vi "server-new.vi"() -> ()   [LabVIEW 2016]
uses:
  <vilib>/rvi/eio/common/nirviEmuClasses.ctl
  <vilib>/rvi/Emulation/niFpgaSctlEmulationGetInTimedLoop.vi
  <vilib>/rvi/Emulation/niFpgaProcessEmulError.vi
  <vilib>/rvi/eio/common/nirviEmuTemplateMethod_errors.vi
  <vilib>/rvi/Emulation/niFpgaEmulationIsFPGAContextNoSignature.vi
  <vilib>/rvi/DataTransferAndStorage/Container/Common/niFpgaContainerGetUniqueNameForEmu.vi
  <vilib>/rvi/Memory/Memory_Emulation/niFpgaMemoryEmulationCacheClearOnFirstRun.vi
  <vilib>/rvi/Memory/Memory_Emulation/nirvimemoryEmulationManagerCache_MakeExclusive.vi
  <vilib>/rvi/Memory/Memory_Emulation/niFpgaMemoryEmulationValidateCache.vi
  <vilib>/rvi/Memory/Memory_Emulation/nirvimemoryEmulationManagerCache_InsertValue.vi
  <vilib>/Utility/error.llb/Clear Errors.vi
  <vilib>/rvi/Memory/Memory_Emulation/nirvimemoryEmulationManagerCache_ReleaseExclusive.vi
  <vilib>/rvi/Memory/Memory_Emulation/nirvimemoryEmulationManagerCache_GetValue.vi
  <vilib>/rvi/Memory/Memory_Emulation/nirvimemoryEmulationManagerCache_SetValue.vi
  <vilib>/rvi/Emulation/niFpgaGetClockAttributes.vi
  <vilib>/rvi/Emulation/niFpgaEmulationReportErrorSimple.vi
  <vilib>/rvi/Emulation/niFpgaCriticalErrorInLSC.vi
  <vilib>/rvi/eio/common/nirviEmuTemplateMethod_noerrors.vi
  <vilib>/rvi/errors/niFpgaSetErrorForExecOnDevCompSimple.vi
  <vilib>/rvi/eio/common/nirviEmuReportErrorAndStop.vi
  <vilib>/rvi/FIFO/Fifo_Resource/nirvififoEmulationSetSize.vi
  <vilib>/rvi/FIFO/Fifo_Resource/nirviFifoEmulationQueueMgr.vi
  <instcachedir>/0/nirviFifoEmulationQueueMgr_E5CAEC123FF24DC58D834DCA3CDAA9B5.lvgen/nirviFifoEmulationQueueMgr_E5CAEC123FF24DC58D834DCA3CDAA9B5_001.vi
  <vilib>/rvi/FIFO/Fifo_Resource/nirvififoEmulationDetermineInputValidOut.vi
  <vilib>/rvi/FIFO/Fifo_Resource/nirvififoEmulationCreateLock.vi
  <vilib>/rvi/FIFO/Fifo_Resource/nirvififoEmulationObtainLock.vi
  <vilib>/rvi/FIFO/Fifo_Resource/nirvififoEmulationReleaseLock.vi
  <vilib>/rvi/occurrence/nirviWaitOnOccurrenceBase.vi
  <vilib>/rvi/errors/nirviReportUnexpectedCaseInternalError.vi
  <vilib>/rvi/errors/nirviReportUnexpectedCaseInternalError (U32).vi
  <vilib>/eio/EIOGrowableMethodNode/genericMethod/EIOGrowableMethodNode.xnode
  <vilib>/rvi/eio/nirviEIOMethodImplementation/nirviEIOMethodImplementation.xnode
  <vilib>/rvi/eio/nirviErrorMerge/nirviErrorMerge.xnode
  <vilib>/rvi/DataTransferAndStorage/Container/XNode/niFpgaContainer.xnode
  <vilib>/rvi/DataTransferAndStorage/Register/Emulation/niFpgaRegisterEmulation.vi
  <vilib>/eio/EIONode/EIONode.xnode
  <vilib>/rvi/FIFO/Fifo_Resource/nirvififoEmulationWrite.vi
panel:
  in  "DO":u32
  in  "Fan Voltage":i16
  out "pas lrms":u32
  out "Temperatures":T1
  out "Sensor Status":u8
  in  "f1":u32
  in  "f0":u32
  in  "Transmit?":bool
  in  "CRDSampData":u32
  in  "Speaker":cluster{"Vscale":fxp<+,32,0>, "Offset":i16}
  in  "Stop":bool
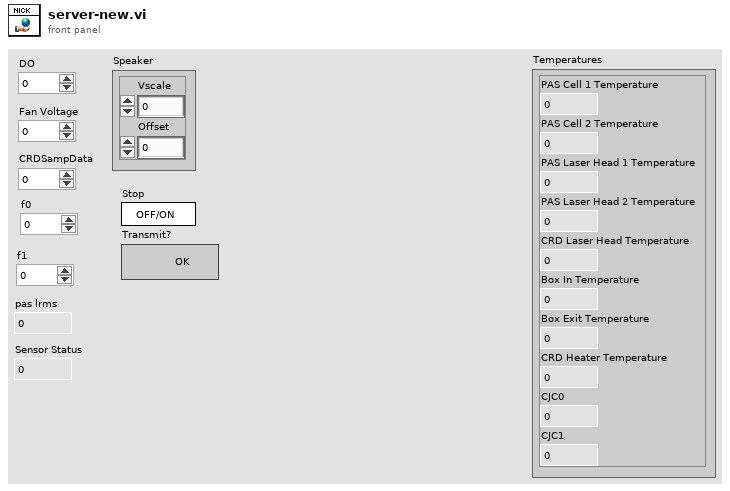
[diagram p1: front panel]
types:
  T1 = cluster{"PAS Cell 1 Temperature":fxp<+/-,24,-2>, "PAS Cell 2 Temperature":fxp<+/-,24,-2>, "PAS Laser Head 1 Temperature":fxp<+/-,24,-2>, "PAS Laser Head 2 Temperature":fxp<+/-,24,-2>, "CRD Laser Head Temperature":fxp<+/-,24,-2>, "Box In Temperature":fxp<+/-,24,-2>, "Box Exit Temperature":fxp<+/-,24,-2>, "CRD Heater Temperature":fxp<+/-,24,-2>, "CJC0":fxp<+/-,24,-2>, "CJC1":fxp<+/-,24,-2>}
  T2 = typedef "nirviEmuClasses.ctl" = enum16{"IO Read", "IO Write", "Method", "Property Read", "Property Write"}
  T3 = cluster{"PAS Cell 1 Temperature":fxp<+/-,24,-2>, "PAS Cell 2 Temperature":fxp<+/-,24,-2>, "PAS Laser Head 1 Temperature":fxp<+/-,24,-2>, "PAS Laser Head 2 Temperature":fxp<+/-,24,-2>, "CRD Laser Head Temperature":fxp<+/-,24,-2>, "Box In Temperature":fxp<+/-,24,-2>, "Box Exit Temperature":fxp<+/-,24,-2>, "CRD Heater Temperature":fxp<+/-,24,-2>, "Mod5/CJC0":fxp<+/-,24,-2>, "Mod5/CJC1":fxp<+/-,24,-2>}
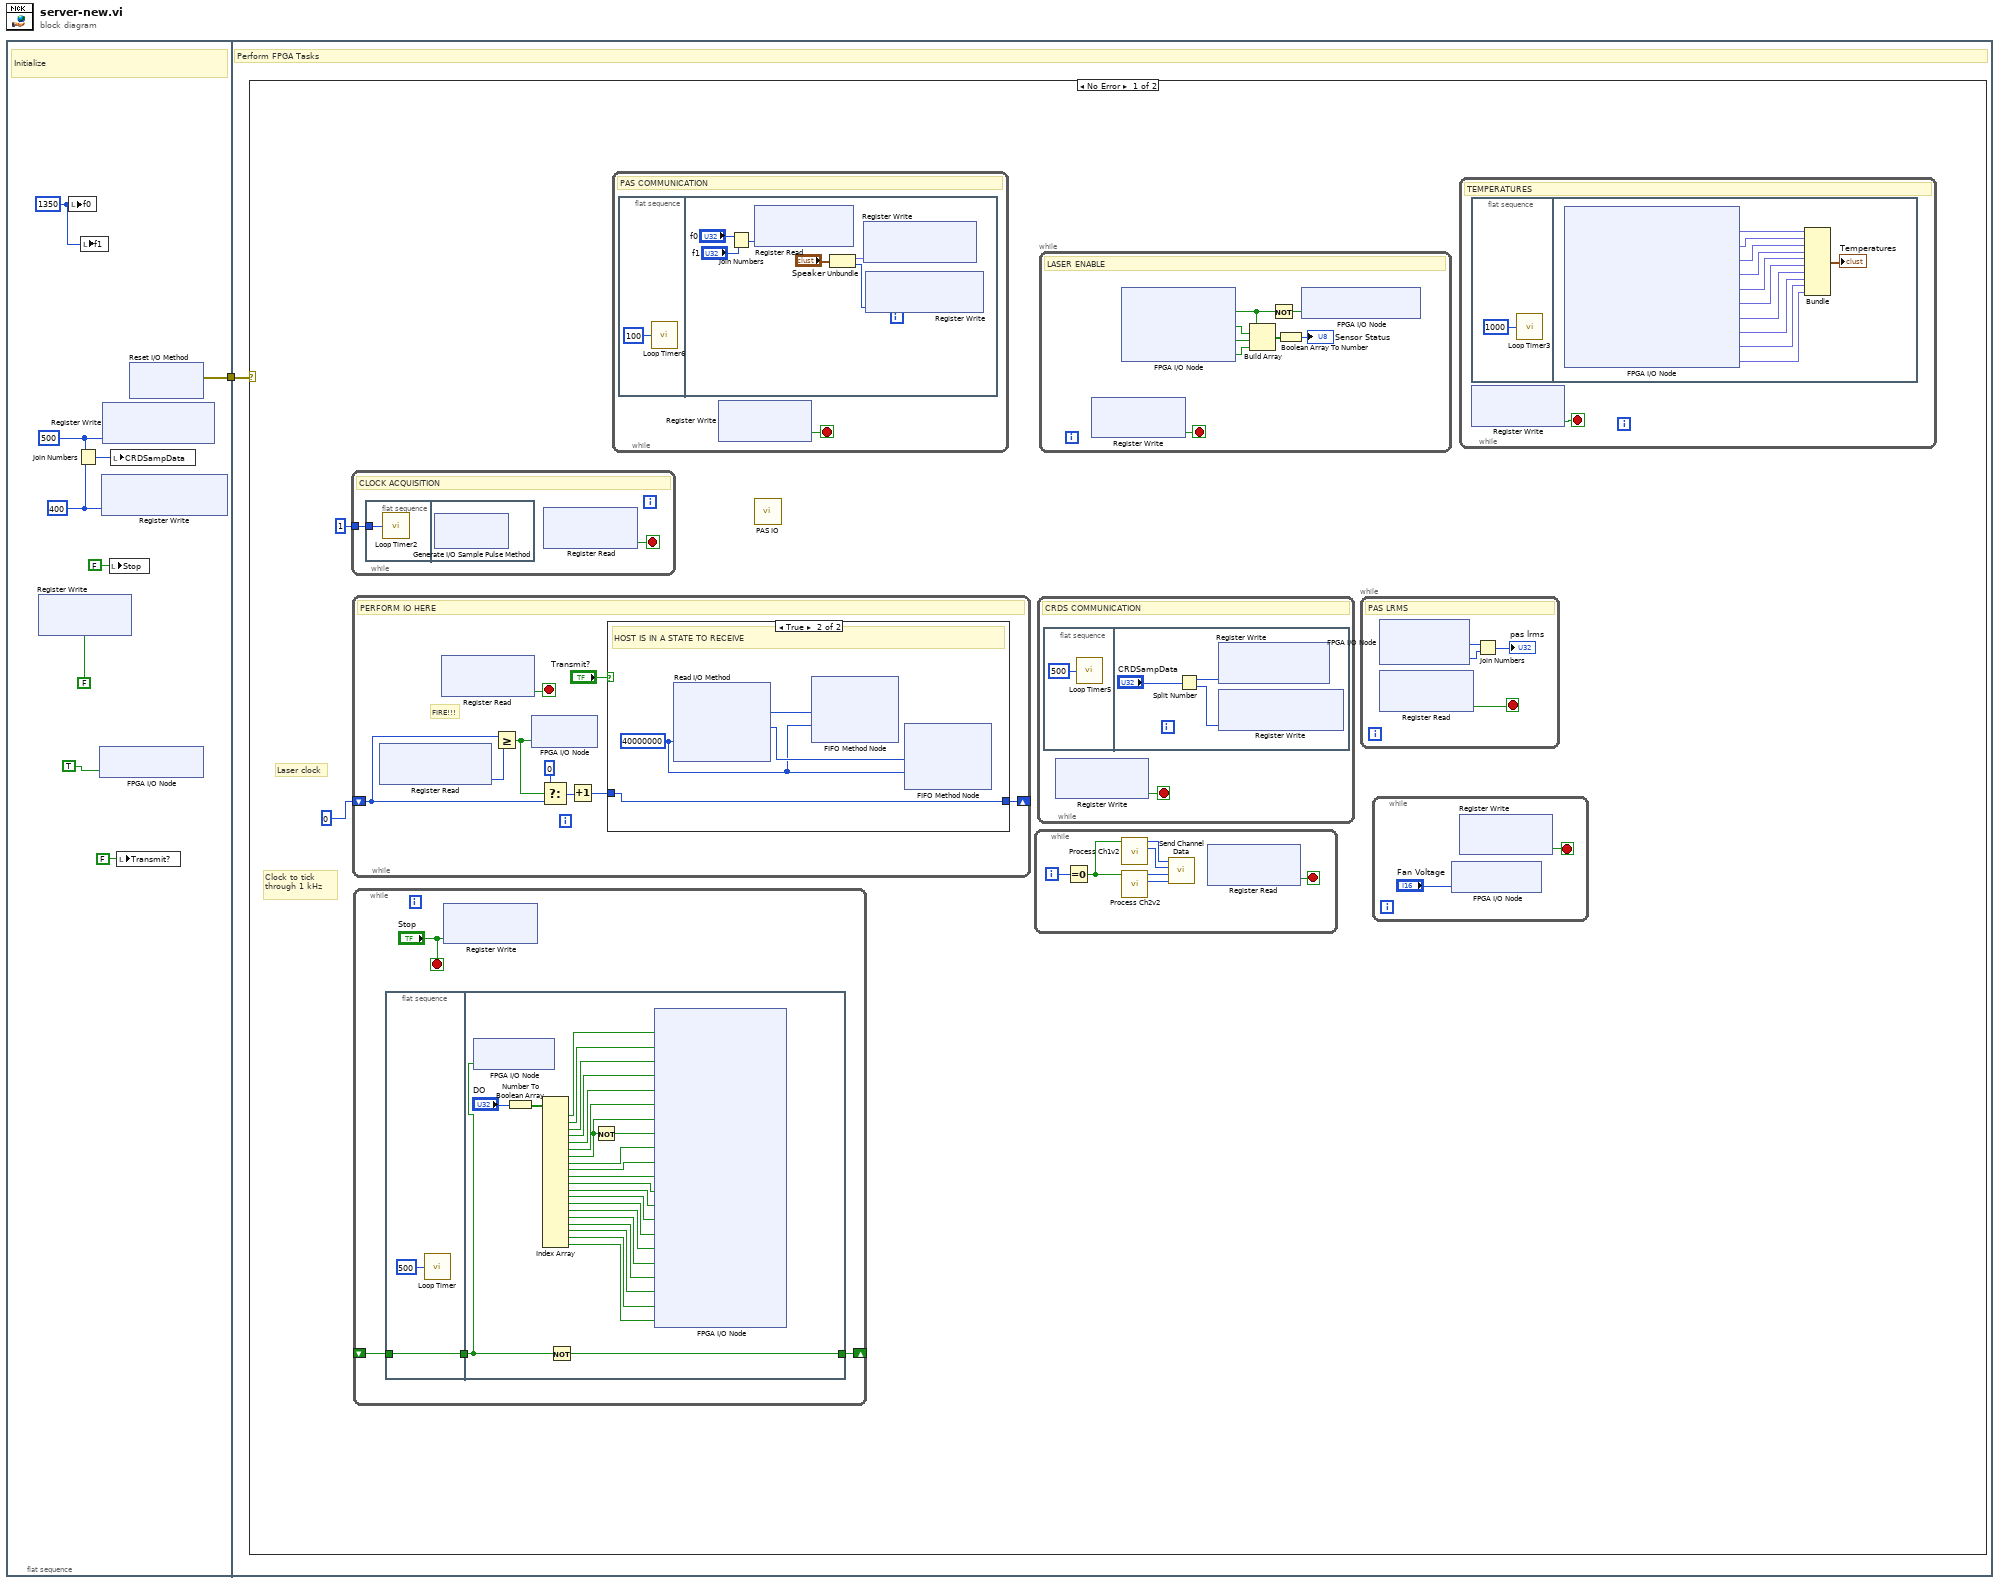
[diagram p0: block diagram]
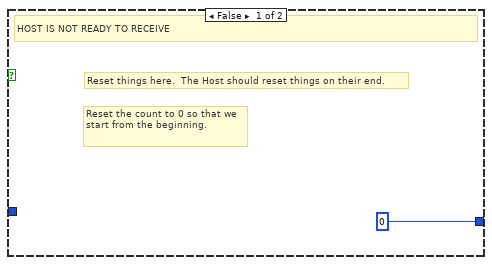
[diagram p2: hidden frame]
diagram:
  n1 = flat-sequence {
    tunnel: [w10] -> w1
    tunnel: w1 -> [w55]
    frame #0 {
      w2 = u32 1350 ("f0")
      w7 = u16 500 ("Data")
      w6 = u16 400 ("Data")
      # "Initialize"
      n2 = xnode ("Register Write")("Data"=FALSE) -> ()  [unwired: 1 in, 1 out]
      n3 = local write "f0"(w2) -> ()
      n4 = Join Numbers(hi=w7, lo=w6) -> ((hi.lo)=w5:u32)
      n5 = local write "f1"(w2) -> ()
      n6 = xnode "FPGA I/O Node"("USB Hub Relay"=TRUE) -> ()  [unwired: 1 in, 1 out]
      n7 = xnode ("Register Write")("Data"=w6) -> ()  [unwired: 1 in, 1 out]
      n8 = xnode ("Register Write")("Data"=w7) -> ()  [unwired: 1 in, 1 out]
      n9 = local write "Stop"(FALSE ("Stop")) -> ()
      n10 = local write "CRDSampData"(w5) -> ()
      n11 = local write "Transmit?"(FALSE ("Transmit?")) -> ()
      n12 = xnode "Reset I/O Method"() -> ("error out"=w10:errorcluster)  [unwired: 2 in, 1 out]
    }
    frame #1 {
      # "Perform FPGA Tasks"
      n13 = case shown="No Error" w55 {
        frame No Error {
          # "Laser clock"
          # "Clock to tick through 1 kHz"
          n14 = while {
            tunnel: u32 1 ("Sample Period (uSec)") -> [w173]
            stop <- w172 stop-if-true
            # "CLOCK ACQUISITION"
            n15 = flat-sequence {
              tunnel: w173 -> [w174]
              frame #0 {
                n16 = call "Loop Timer2"("Count(uSec)"=w174) -> ()  [unwired: 1 out]
              }
              frame #1 {
                n17 = xnode "Generate I/O Sample Pulse Method"() -> ()  [unwired: 2 in, 2 out]
              }
            }
            n18 = xnode ("Register Read")() -> ("Data"=w172:bool)  [unwired: 1 in, 1 out]
          }
          n19 = while {
            shift-right: [w89] -> _
            shift-left: u16 0 ("Number of Samples") -> [w90]
            stop <- w84 stop-if-true
            # "FIRE!!!"
            # "PERFORM IO HERE"
            n20 = xnode ("Register Read")() -> ("Data"=w86:u16)  [unwired: 1 in, 1 out]
            n21 = xnode ("Register Read")() -> ("Data"=w84:bool)  [unwired: 1 in, 1 out]
            n22 = Greater Or Equal?(x=w90, y=w86) -> (x >= y?=w91:bool)
            n23 = xnode "FPGA I/O Node"("CRDS"=w91) -> ()  [unwired: 1 in, 1 out]
            n24 = Select(t=u16 0 ("Number of Samples"), s=w91, f=w90) -> (s? t:f=w88:u16)
            n25 = Increment(x=w88) -> (x+1=w87:u16)
            n26 = case shown="True" "Transmit?" {
              tunnel: w87 -> [_ w97]
              tunnel: [u16 0 ("Number of Samples") w97] -> w89
              frame False {
                # "Reset things here.  The Host should reset things on their end."
                # "Reset the count to 0 so that we start from the beginning."
                # "HOST IS NOT READY TO RECEIVE"
              }
              frame True {
                w94 = 40000000 ("Timeout")
                # "HOST IS IN A STATE TO RECEIVE"
                n27 = xnode "Read I/O Method"("Timeout"=w94) -> ("CRD Las Ch 1"=w96:i16, "CRD Las Ch 2"=w95:i16)  [unwired: 3 in, 4 out]
                n28 = xnode ("FIFO Method Node")("Element"=w96, "Timeout"=w94) -> ()  [unwired: 2 in, 3 out]
                n29 = xnode ("FIFO Method Node")("Element"=w95, "Timeout"=w94) -> ()  [unwired: 2 in, 3 out]
              }
            }
          }
          n30 = while {
            shift-right: [w197] -> _
            shift-left: _ -> [w196]
            stop <- "Stop" stop-if-true
            n31 = flat-sequence {
              tunnel: w196 -> [w199]
              tunnel: [w199] -> w194
              tunnel: [w224] -> w197
              tunnel: w194 -> [w223]
              frame #0 {
                n32 = call "Loop Timer"("Count(mSec)"=u32 500) -> ()  [unwired: 1 out]
              }
              frame #1 {
                n33 = xnode "FPGA I/O Node"("Heartbeat"=w223) -> ()  [unwired: 1 in, 1 out]
                n34 = Number To Boolean Array(number="DO") -> (Boolean array=w221:bool[])
                n35 = Index Array(array=w221) -> (element #1=w220:bool, element #2=w219:bool, element #3=w218:bool, element #4=w217:bool, element #5=w216:bool, element #6=w215:bool, element #7=w214:bool, element #8=w212:bool, element #9=w211:bool, element #10=w210:bool, element #11=w209:bool, element #12=w208:bool, element #13=w207:bool, element #14=w206:bool, element #15=w205:bool, element #16=w204:bool, element #17=w203:bool, element #18=w202:bool, element #19=w201:bool, element #20=w200:bool)  [unwired: 20 in]
                n36 = Not(x=w223) -> (.not. x?=w224:bool)
                n37 = Not(x=w214) -> (.not. x?=w213:bool)
                n38 = xnode "FPGA I/O Node"("PAS Laser Relay 1"=w220, "PAS Heater 1"=w219, "PAS Heater 2"=w218, "PAS Laser Relay 2"=w217, "PAS Speaker Enable 1"=w216, "PAS Speaker Enable 2"=w215, "hb 1 ctl 1"=w214, "hb 1 ctl 2"=w213, "Fan Enable"=w212, "CRD Laser Enable"=w211, "CRD Heater Enable"=w210, "Vacuum Pump"=w209, "AC Spare"=w208, "uv light enable"=w207, "Solenoid Relay 1"=w206, "Solenoid Relay 2"=w205, "Spare DC Relay 1"=w204, "USB Hub Relay"=w203, "Spare DC Relay 2"=w202, "FP Aux 1"=w201, "FP Aux 2"=w200) -> ()  [unwired: 21 in, 21 out]
              }
            }
            n39 = xnode ("Register Write")("Data"="Stop") -> ()  [unwired: 1 in, 1 out]
          }
          n40 = while {
            stop <- w181 stop-if-true
            # "PAS COMMUNICATION"
            n41 = flat-sequence {
              frame #0 {
                n42 = call "Loop Timer6"("Count(mSec)"=u32 100) -> ()  [unwired: 1 out]
              }
              frame #1 {
                n43 = Join Numbers(hi="f0", lo="f1") -> ((hi.lo)=w183:u64)
                n44 = xnode ("Register Read")("Data"=w183) -> ()  [unwired: 1 in, 1 out]
                n45 = Unbundle("Speaker") -> ("Vscale"=w188:fxp<+,32,0>, "Offset"=w187:i16)
                n46 = xnode ("Register Write")("Data"=w188) -> ()  [unwired: 1 in, 1 out]
                n47 = xnode ("Register Write")("Data"=w187) -> ()  [unwired: 1 in, 1 out]
              }
            }
            n48 = xnode ("Register Write")() -> ("Data"=w181:bool)  [unwired: 1 in, 1 out]
          }
          n49 = call "PAS IO.vi"() -> ()  [unwired: 20 in]
          n50 = while {
            i -> [w78]
            stop <- w79 stop-if-true
            n51 = Equal To 0?(x=w78) -> (x = 0?=w77:bool)
            n52 = call "Process Ch1v2.vi"("Init?"=w77) -> ("Max1"=w82:u32, "Max0"=w83:u32)  [unwired: 9 in]
            n53 = call "Process Ch2v2.vi"("Init?"=w77) -> ("Max1"=w80:u32, "Max0"=w81:u32)  [unwired: 9 in]
            n54 = call "Send Channel Data.vi"("Max3"=w80, "Max2"=w81, "Max1"=w82, "Max0"=w83) -> ()  [unwired: 8 in]
            n55 = xnode ("Register Read")() -> ("Data"=w79:bool)  [unwired: 1 in, 1 out]
          }
          n56 = while {
            stop <- w189 stop-if-true
            # "CRDS COMMUNICATION"
            n57 = flat-sequence {
              frame #0 {
                n58 = call "Loop Timer5"("Count(mSec)"=u32 500) -> ()  [unwired: 1 out]
              }
              frame #1 {
                n59 = Split Number(x="CRDSampData") -> (hi(x)=w192:u16, lo(x)=w193:u16)
                n60 = xnode ("Register Write")("Data"=w192) -> ()  [unwired: 1 in, 1 out]
                n61 = xnode ("Register Write")("Data"=w193) -> ()  [unwired: 1 in, 1 out]
              }
            }
            n62 = xnode ("Register Write")() -> ("Data"=w189:bool)  [unwired: 1 in, 1 out]
          }
          n63 = while {
            stop <- w171 stop-if-true
            # "LASER ENABLE"
            n64 = xnode ("Register Write")() -> ("Data"=w171:bool)  [unwired: 1 in, 1 out]
            n65 = xnode "FPGA I/O Node"() -> ("Interlock Sense"=w165:bool, "hb 1 status 1"=w169:bool, "hb 1 status 2"=w168:bool, "Soft Power Down"=w167:bool)  [unwired: 4 in, 4 out]
            n66 = Build Array(w165, w169, w168, w167) -> (w166:bool[])
            n67 = Not(x=w165) -> (.not. x?=w164:bool)
            n68 = Boolean Array To Number(Boolean array=w166) -> (number=→"Sensor Status":u8)
            n69 = xnode "FPGA I/O Node"("Interlock Indicator"=w164) -> ()  [unwired: 1 in, 1 out]
          }
          n70 = while {
            stop <- w63 stop-if-true
            # "PAS LRMS"
            n71 = xnode "FPGA I/O Node"() -> ("PAS LRMS 1"=w62:i16, "PAS LRMS 2"=w61:i16)  [unwired: 2 in, 2 out]
            n72 = xnode ("Register Read")() -> ("Data"=w63:bool)  [unwired: 1 in, 1 out]
            n73 = Join Numbers(hi=w62, lo=w61) -> ((hi.lo)=→"pas lrms":u32)
          }
          n74 = while {
            stop <- w59 stop-if-true
            n75 = xnode "FPGA I/O Node"("Fan Voltage"="Fan Voltage") -> ()  [unwired: 1 in, 1 out]
            n76 = xnode ("Register Write")() -> ("Data"=w59:bool)  [unwired: 1 in, 1 out]
          }
          n77 = while {
            stop <- w64 stop-if-true
            # "TEMPERATURES"
            n78 = flat-sequence {
              frame #0 {
                n79 = call "Loop Timer3"("Count(mSec)"=u32 1000 ("Sample Period (uSec)")) -> ()  [unwired: 1 out]
              }
              frame #1 {
                n80 = xnode "FPGA I/O Node"() -> ("PAS Cell 1 Temperature"=w76:fxp<+/-,24,-2>, "PAS Cell 2 Temperature"=w75:fxp<+/-,24,-2>, "PAS Laser Head 1 Temperature"=w74:fxp<+/-,24,-2>, "PAS Laser Head 2 Temperature"=w73:fxp<+/-,24,-2>, "CRD Laser Head Temperature"=w72:fxp<+/-,24,-2>, "Box In Temperature"=w71:fxp<+/-,24,-2>, "Box Exit Temperature"=w70:fxp<+/-,24,-2>, "CRD Heater Temperature"=w69:fxp<+/-,24,-2>, "Mod5/CJC0"=w68:fxp<+/-,24,-2>, "Mod5/CJC1"=w67:fxp<+/-,24,-2>)  [unwired: 10 in, 10 out]
                n81 = Bundle("PAS Cell 1 Temperature"=w76, "PAS Cell 2 Temperature"=w75, "PAS Laser Head 1 Temperature"=w74, "PAS Laser Head 2 Temperature"=w73, "CRD Laser Head Temperature"=w72, "Box In Temperature"=w71, "Box Exit Temperature"=w70, "CRD Heater Temperature"=w69, "Mod5/CJC0"=w68, "Mod5/CJC1"=w67) -> (→"Temperatures":T3)  [unwired: 1 in]
              }
            }
            n82 = xnode ("Register Write")() -> ("Data"=w64:bool)  [unwired: 1 in, 1 out]
          }
        }
        frame Error {
        }
      }
    }
  }
